vi "Is Allowed Path.vi"(10 "Data Cluster in":T1, 11 "Path":path) -> (3 "Boolean":bool)   [LabVIEW 2025, in "Scripting Server.lvlib"]
uses:
  Scripting Server.lvlib
  Config Data.ctl
  Module Data--cluster.ctl
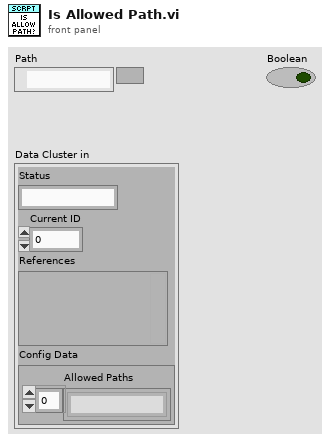
[diagram p1: front panel]
types:
  T1 = typedef "Scripting Server.lvlib/Module Data--cluster.ctl" = cluster{"Status":string, "Current ID":i32, "References":variant, "Config Data":T2}
  T2 = typedef "Scripting Server.lvlib/Config Data.ctl" = cluster{"Allowed Paths":string[]}
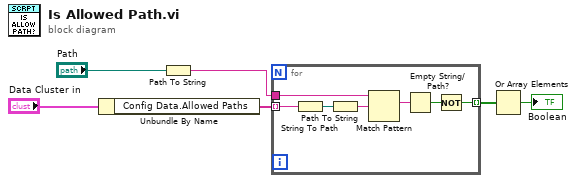
[diagram p0: block diagram]
diagram:
  n1 = Unbundle By Name("Data Cluster in") -> ("Config Data.Allowed Paths"=w6:string[])
  n2 = Path To String(path="Path") -> (string=w2:string)
  n3 = for {
    tunnel: w2 -> [w13]
    tunnel: w6 -> [w7] mode=indexing
    tunnel: [w8] -> w4 mode=indexing
    n4 = String To Path(string=w7) -> (path=w12:path)
    n5 = Path To String(path=w12) -> (string=w11:string)
    n6 = Match Pattern(string=w13, regular expression=w11) -> (match substring=w10:string)  [unwired: 1 in, 3 out]
    n7 = Empty String/Path?(string/path=w10) -> (empty?=w9:bool)
    n8 = Not(x=w9) -> (.not. x?=w8:bool)
  }
  n9 = Or Array Elements(Boolean array=w4) -> (logical OR=→"Boolean":bool)
